vi "Create Workbook and set cell value.vi"() -> ()   [LabVIEW 2013]
uses:
  Typedefs/Worksheet Format.ctl
  Data/Polymorphic VIs/Set Cell (String).vi
panel:
  in  "Worksheet Format (XLSX)":T1
  in  "Row (0)":i32
  in  "Value":string
  in  "Column (0)":i32
  in  "Sheetname (Sheet1)":string="Sheet1"
  in  "File Name":path=path "C:/PhaeronGit/LVNPOI/Scratch/test.xls"
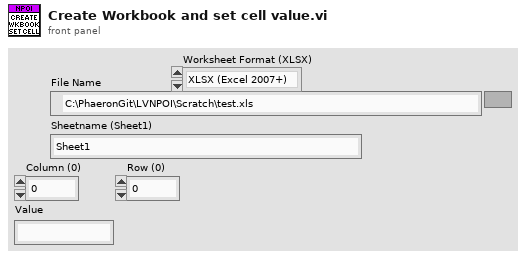
[diagram p1: front panel]
types:
  T1 = typedef "Worksheet Format.ctl" = enum16{"XLSX (Excel 2007+)", "XLS (Excel Legacy)"}
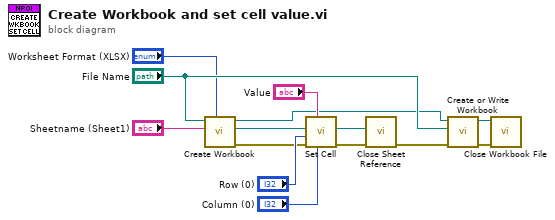
[diagram p0: block diagram]
diagram:
  n1 = call "Create Workbook.vi"("Worksheet Format (XLSX)"="Worksheet Format (XLSX)", "Sheetname (Sheet1)"="Sheetname (Sheet1)", "File Name"="File Name") -> ("error out"=w1:errorcluster, "Sheet Reference"=w3:refnum<k24>, "IWorkbook Reference"=w2:refnum<k24>)  [unwired: 6 in]
  n2 = call-poly "Set Cell.vi"("Column"="Column (0)", "Value"="Value", "error in (no error)"=w1, "Row"="Row (0)", "Sheet Reference"=w3) -> ("error out"=w10:errorcluster, "Sheet Reference out"=w11:refnum<k24>)  [unwired: 5 in]
  n3 = call "Close Sheet Reference.vi"("error in (no error)"=w10, "Sheet Reference"=w11) -> ("error out"=w14:errorcluster)  [unwired: 9 in]
  n4 = call "Create or Write Workbook.vi"("error in (no error)"=w14, "File Name"="File Name", "IWorkbook Reference"=w2) -> ("error out"=w13:errorcluster, "IWorkbook Reference Out"=w12:refnum<k24>)  [unwired: 7 in]
  n5 = call "Close Workbook File.vi"("error in (no error)"=w13, "IWorkbook Reference"=w12) -> ()  [unwired: 9 in, 1 out]
